vi "VI Tree.vi"   [LabVIEW 2013, in "AWG.lvlib" / "Agilent 33XXX Series.lvlib"]
doc: "This is the instrument driver for the Agilent 33XXX Series. The VI Tree displays all the user-callable VIs of the instrument driver in an organized table."
uses:
  Agilent 33XXX Series.lvlib
  Configure/Configure Modulation (Pulse Width).vi
panel:
  # "(c) 2005 -2013  National Instruments.  ALL RIGHTS RESERVED."
  # "SEE DIAGRAM\nFOR VI TREE."
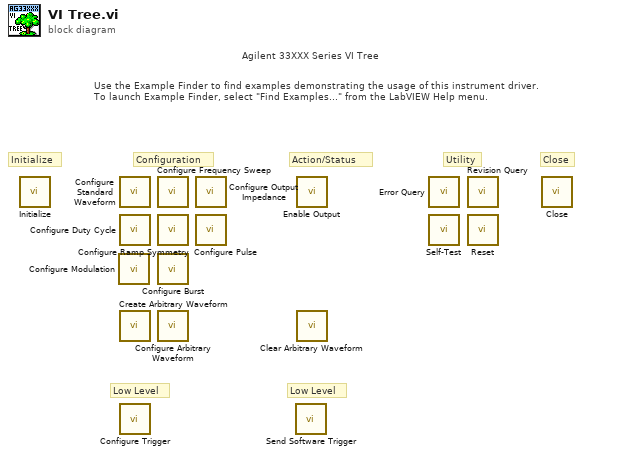
[diagram p0: block diagram]
diagram:
  # "Agilent 33XXX Series VI Tree"
  # "Low Level"
  # "Low Level"
  # "Use the Example Finder to find examples demonstrating the usage of this instrument driver.\nTo launch Example Finder, select \"Find Examples...\" from the LabVIEW Help menu."
  # "Configuration"
  # "Utility"
  # "Action/Status"
  # "Close"
  # "Initialize"
  n1 = call "Initialize.vi"() -> ()  [unwired: 9 in, 3 out]
  n2 = call-poly "Configure Modulation.vi"() -> ()  [unwired: 14 in, 2 out]
  n3 = call "Configure Standard Waveform.vi"() -> ()  [unwired: 10 in, 2 out]
  n4 = call "Configure Duty Cycle.vi"() -> ()  [unwired: 10 in, 2 out]
  n5 = call "Create Arbitrary Waveform.vi"() -> ()  [unwired: 10 in, 2 out]
  n6 = call "Configure Trigger.vi"() -> ()  [unwired: 10 in, 2 out]
  n7 = call "Configure Frequency Sweep.vi"() -> ()  [unwired: 10 in, 2 out]
  n8 = call "Configure Ramp Symmetry.vi"() -> ()  [unwired: 10 in, 2 out]
  n9 = call "Configure Burst.vi"() -> ()  [unwired: 10 in, 2 out]
  n10 = call "Configure Arbitrary Waveform.vi"() -> ()  [unwired: 10 in, 2 out]
  n11 = call "Configure Output Impedance.vi"() -> ()  [unwired: 10 in, 2 out]
  n12 = call "Configure Pulse.vi"() -> ()  [unwired: 10 in, 2 out]
  n13 = call "Send Software Trigger.vi"() -> ()  [unwired: 10 in, 2 out]
  n14 = call "Enable Output.vi"() -> ()  [unwired: 10 in, 2 out]
  n15 = call "Clear Arbitrary Waveform.vi"() -> ()  [unwired: 10 in, 2 out]
  n16 = call "Error Query.vi"() -> ()  [unwired: 8 in, 4 out]
  n17 = call "Self-Test.vi"() -> ()  [unwired: 8 in, 4 out]
  n18 = call "Revision Query.vi"() -> ()  [unwired: 8 in, 4 out]
  n19 = call "Reset.vi"() -> ()  [unwired: 10 in, 2 out]
  n20 = call "Close.vi"() -> ()  [unwired: 11 in, 1 out]
